vi "Compose.vi"(8 "error in":errorcluster, 10 "Orient3d 2":refnum<class "Orient3d.lvclass">, 11 "Orient3d 1":refnum<class "Orient3d.lvclass">) -> (0 "error out":errorcluster, 3 "Orient3d out":refnum<class "Orient3d.lvclass">)   [LabVIEW 2023, in "Orient3d.lvclass"]
uses:
  Orient3d.lvclass
  <vilib>/Analysis/baseanly.llb/Real A x B.vi
  <vilib>/Analysis/NI_AALBase.lvlib
panel:
  # "Result is rotation Orient3d 1 followed by Orient3d 2"
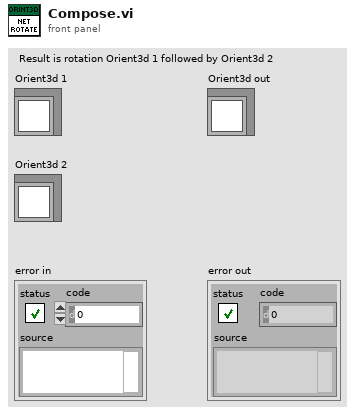
[diagram p1: front panel]
types:
  T1 = typedef "NI_Matrix.lvlib/RealMatrix.ctl" = dbl[][]
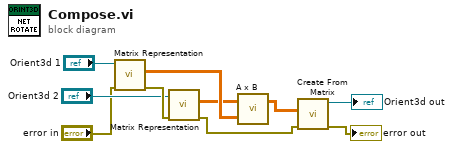
[diagram p0: block diagram]
diagram:
  n1 = call "Matrix Representation.vi"("error in"="error in", "Orient3d in"="Orient3d 1") -> ("error out"=w9:errorcluster, "Rotation Matrix"=w7:T1)  [unwired: 7 in, 1 out]
  n2 = call "Matrix Representation.vi"("error in"=w9, "Orient3d in"="Orient3d 2") -> ("error out"=w3:errorcluster, "Rotation Matrix"=w6:T1)  [unwired: 7 in, 1 out]
  n3 = call-poly <vilib>:"A x B.vi"("B"=w7, "A"=w6) -> ("A x B"=w4:T1)  [unwired: 1 out]
  n4 = call "Create From Matrix.vi"("error in"=w3, "Rotation Matrix"=w4) -> ("error out"=→"error out":errorcluster, "Orient3d out"=→"Orient3d out":refnum<class "Orient3d.lvclass">)  [unwired: 8 in]
